vi "Emballage_BDD_ON_OFF_Lecteur.vi"(8 "Error in":errorcluster caption="Error in (no error)", 10 "TimeOut (sec)":dbl=5.0 format="%#_13g", 11 "ON/OFF lecteur":T1=enum."OFF") -> (0 "Error out":errorcluster, 2 "TIMEOUT_FIN?":bool, 3 "Etiquette scanné":string)   [LabVIEW 2020]
uses:
  enum_ON_OFF_Lecteur.ctl
  Modules/FS/60_FS_Controles/60_FS_SetGet.ctl
panel:
  out "vide ?":bool
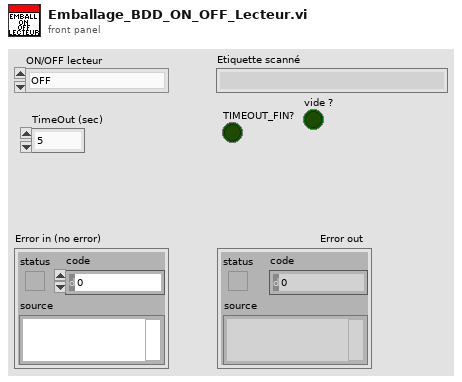
[diagram p1: front panel]
types:
  T1 = typedef "enum_ON_OFF_Lecteur.ctl" = enum16{"ON_COURT", "OFF", "ON", "OFF (open/Close)", "ON (open/close)"}
  T2 = typedef "60_FS_SetGet.ctl" = enum16{"set", "get"}
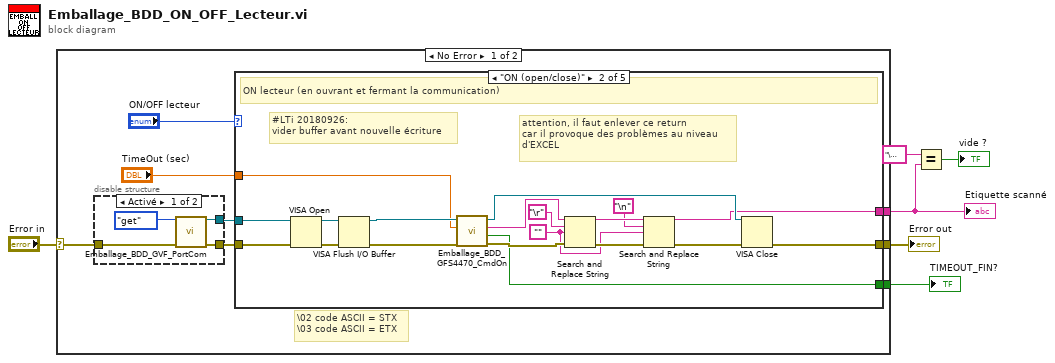
[diagram p0: block diagram]
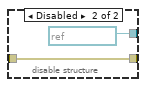
[diagram p2: hidden frame]
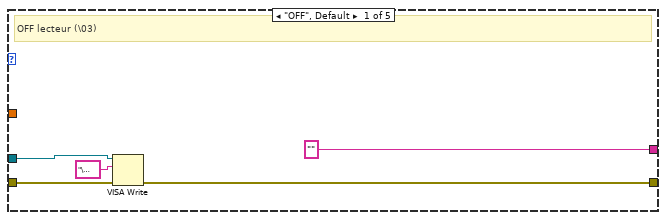
[diagram p3: hidden frame]
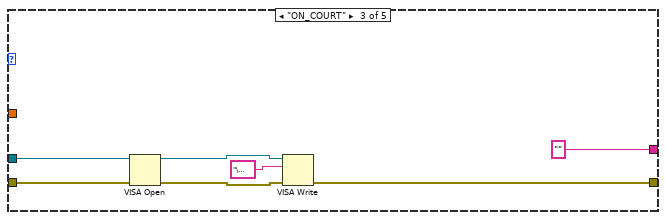
[diagram p4: hidden frame]
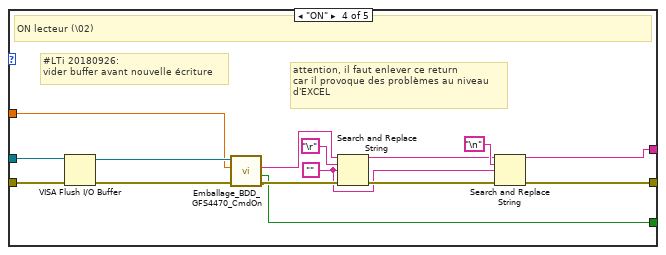
[diagram p5: hidden frame]
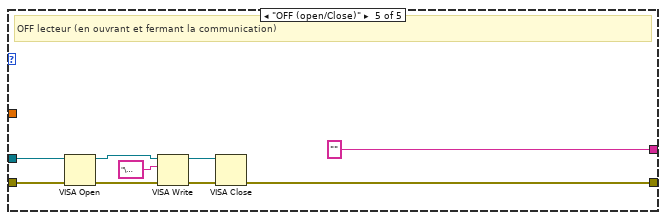
[diagram p6: hidden frame]
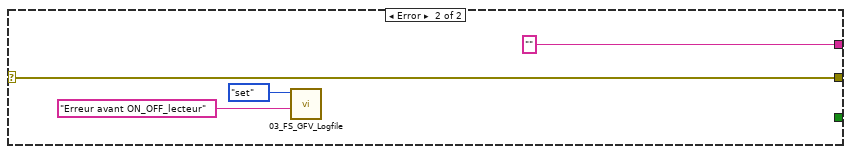
[diagram p7: hidden frame]
diagram:
  n1 = case shown="No Error" "Error in" {
    selector: "Error in" -> [w13 w79]
    tunnel: [w12 w79] -> w5
    tunnel: [w10 "" ("result string")] -> w3
    tunnel: [w8 _] -> w4
    frame No Error {
      # "\\02 code ASCII = STX\n\\03 code ASCII = ETX"
      n2 = disable-structure shown="Activé" {
        disable-tunnel: w13 -> [w18 w19]
        disable-tunnel: [w17 w19] -> w11
        disable-tunnel: [w16 refnum<visa-resource-name> "COM23" ("PortCom Scanner")] -> w9
        frame Enabled {
          n3 = call "Emballage_BDD_GVF_PortCom.vi"("Énum"=enum16{"get", "set"}."get", "Error in"=w18) -> ("PortCom Scanner"=w16:refnum<visa-resource-name>, "Error out"=w17:errorcluster)  [unwired: 7 in, 5 out]
        }
        frame Disabled {
        }
      }
      n4 = case shown="\"ON (open/close)\"" "ON/OFF lecteur" {
        tunnel: [w24 w42 w47 w56 w69] -> w12
        tunnel: w11 -> [w23 w44 w48 w64 w74]
        tunnel: w9 -> [w22 w43 w46 w65 w73]
        tunnel: ["" ("result string") w29 "" ("result string") w54 "" ("result string")] -> w10
        tunnel: [_ w34 _ w59 _] -> w8
        tunnel: "TimeOut (sec)" -> [_ w26 _ w52 _]
        frame "OFF", Default {
          # "OFF lecteur (\\03)"
          n5 = VISA Write(VISA resource name=w22, write buffer="\u0003", error in (no error)=w23) -> (error out=w24:errorcluster)  [unwired: 2 out]
        }
        frame "ON (open/close)" {
          w28 = ""
          # "#LTi 20180926:\nvider buffer avant nouvelle écriture"
          # "attention, il faut enlever ce return\ncar il provoque des problèmes au niveau\nd'EXCEL"
          # "ON lecteur (en ouvrant et fermant la communication)"
          n6 = VISA Open(error in (no error)=w44, VISA resource name=w43) -> (VISA resource name=w41:refnum<visa-resource-name>, error out=w40:errorcluster)  [unwired: 3 in]
          n7 = VISA Flush I/O Buffer(VISA resource name=w41, error in (no error)=w40) -> (VISA resource name out=w39:refnum<visa-resource-name>, error out=w38:errorcluster)  [unwired: 1 in]
          n8 = call "Emballage_BDD_GFS4470_CmdOn.vi"("error in (no error)"=w38, "TimeOut (sec)"=w26, "VISA Datalogic 5"=w39) -> ("sortie d'erreur"=w35:errorcluster, "TIMEOUT_FIN?"=w34:bool, "buffer de lecture"=w36:string, "Nom de ressource VISA en sortie"=w37:refnum<visa-resource-name>)  [unwired: 5 in]
          n9 = Search and Replace String(input string=w36, search string="\r", replace string=w28, error in=w35) -> (result string=w30:string, error out=w32:errorcluster)  [unwired: 4 in, 2 out]
          n10 = Search and Replace String(input string=w30, search string="\n", replace string=w28, error in=w32) -> (result string=w29:string, error out=w31:errorcluster)  [unwired: 4 in, 2 out]
          n11 = VISA Close(VISA resource name=w37, error in (no error)=w31) -> (error out=w42:errorcluster)
        }
        frame "ON_COURT" {
          n12 = VISA Open(error in (no error)=w48, VISA resource name=w46) -> (VISA resource name=w50:refnum<visa-resource-name>, error out=w49:errorcluster)  [unwired: 3 in]
          n13 = VISA Write(VISA resource name=w50, write buffer="\u0002", error in (no error)=w49) -> (error out=w47:errorcluster)  [unwired: 2 out]
        }
        frame "ON" {
          w55 = ""
          # "#LTi 20180926:\nvider buffer avant nouvelle écriture"
          # "attention, il faut enlever ce return\ncar il provoque des problèmes au niveau\nd'EXCEL"
          # "ON lecteur (\\02)"
          n14 = VISA Flush I/O Buffer(VISA resource name=w65, error in (no error)=w64) -> (VISA resource name out=w62:refnum<visa-resource-name>, error out=w63:errorcluster)  [unwired: 1 in]
          n15 = call "Emballage_BDD_GFS4470_CmdOn.vi"("error in (no error)"=w63, "TimeOut (sec)"=w52, "VISA Datalogic 5"=w62) -> ("sortie d'erreur"=w60:errorcluster, "TIMEOUT_FIN?"=w59:bool, "buffer de lecture"=w61:string)  [unwired: 5 in, 1 out]
          n16 = Search and Replace String(input string=w61, search string="\r", replace string=w55, error in=w60) -> (result string=w53:string, error out=w57:errorcluster)  [unwired: 4 in, 2 out]
          n17 = Search and Replace String(input string=w53, search string="\n", replace string=w55, error in=w57) -> (result string=w54:string, error out=w56:errorcluster)  [unwired: 4 in, 2 out]
        }
        frame "OFF (open/Close)" {
          # "OFF lecteur (en ouvrant et fermant la communication)"
          n18 = VISA Open(error in (no error)=w74, VISA resource name=w73) -> (VISA resource name=w72:refnum<visa-resource-name>, error out=w71:errorcluster)  [unwired: 3 in]
          n19 = VISA Write(VISA resource name=w72, write buffer="\u0003", error in (no error)=w71) -> (VISA resource name out=w68:refnum<visa-resource-name>, error out=w70:errorcluster)  [unwired: 1 out]
          n20 = VISA Close(VISA resource name=w68, error in (no error)=w70) -> (error out=w69:errorcluster)
        }
      }
    }
    frame Error {
      n21 = call "03_FS_GFV_Logfile.vi"("Chaîne"="Erreur avant ON_OFF_lecteur", "States"=60_FS_SetGet."set") -> ()  [unwired: 8 in, 2 out]
    }
  }
  "Error out" <- w5
  "Etiquette scanné" <- w3
  "TIMEOUT_FIN?" <- w4
  n22 = Equal?(x="\u0002\u0018", y=w3) -> (x = y?=→"vide ?":bool)
